vi "Reclosing.vi"(5 "Recloser Settings":T1, 6 "Counter In":dbl, 8 "Reclose In":bool, 9 "RMS values":dbl[](array[numeric]), 10 "PLL output":cluster{dbl, dbl[], dbl, dbl[]}, 11 "Reclose?":bool) -> (0 "Phase difference":dbl, 1 "frequency difference":dbl, 2 "magnitude difference":dbl, 3 "Recloser action":bool, 4 "Counter Out":dbl)   [LabVIEW 2016]
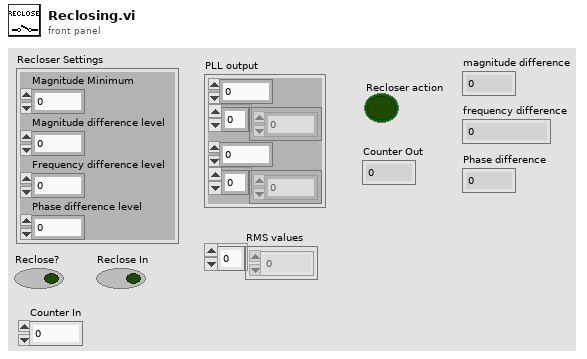
[diagram p1: front panel]
types:
  T1 = cluster{"Magnitude Minimum":dbl, "Magnitude difference level":dbl, "Frequency difference level":dbl, "Phase difference level":dbl}
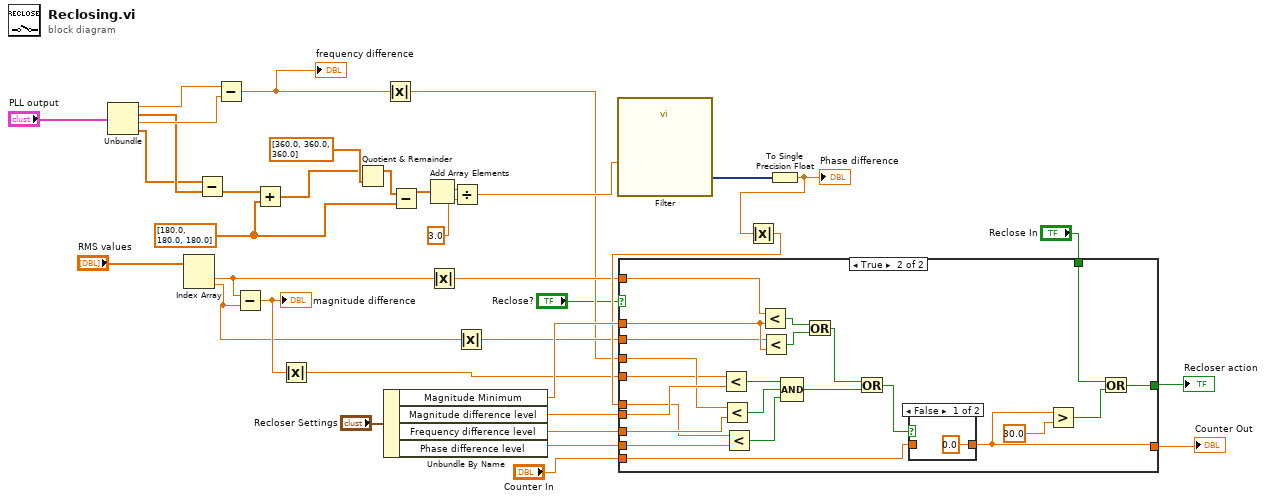
[diagram p0: block diagram]
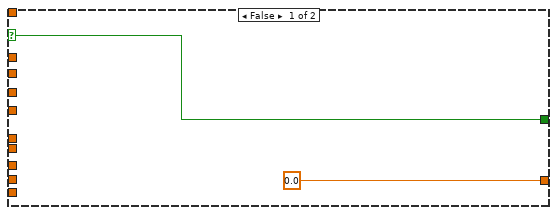
[diagram p2: hidden frame]
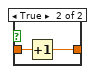
[diagram p3: hidden frame]
diagram:
  w26 = dbl[] [180.0, 180.0, 180.0] ("y")
  n1 = Unbundle("PLL output") -> (w14:dbl, w12:dbl[], w13:dbl, w11:dbl[])
  n2 = Index Array(array="RMS values") -> (element #1=w8:dbl, element #2=w7:dbl)  [unwired: 2 in]
  n3 = Subtract(x=w11, y=w12) -> (x-y=w36:dbl[])
  n4 = Subtract(x=w14, y=w13) -> (x-y=w10:dbl)
  "frequency difference" <- w10
  n5 = Subtract(x=w8, y=w7) -> (x-y=w20:dbl)
  "magnitude difference" <- w20
  n6 = Add(x=w36, y=w26) -> (x+y=w29:dbl[])
  n7 = Absolute Value(x=w20) -> (abs(x)=w2:dbl)
  n8 = Quotient & Remainder(x=w29, y=dbl[] [360.0, 360.0, 360.0]) -> (x-y*floor(x/y)=w32:dbl[])  [unwired: 1 out]
  n9 = Unbundle By Name("Recloser Settings") -> ("Magnitude Minimum"=w25:dbl, "Magnitude difference level"=w24:dbl, "Frequency difference level"=w23:dbl, "Phase difference level"=w22:dbl)
  n10 = Absolute Value(x=w10) -> (abs(x)=w16:dbl)
  n11 = Subtract(x=w32, y=w26) -> (x-y=w31:dbl[])
  n12 = Add Array Elements(numeric array=w31) -> (sum=w35:dbl)
  n13 = Absolute Value(x=w8) -> (abs(x)=w17:dbl)
  n14 = Divide(x=w35, y=3.0 ("x")) -> (x/y=w27:dbl)
  n15 = Absolute Value(x=w7) -> (abs(x)=w18:dbl)
  n16 = call "Filter"("Signal"=w27) -> ("Filtered Signal"=w30:dynamicdata)  [unwired: 9 in, 1 out]
  n17 = To Single Precision Float(number=w30) -> (single precision float=w21:sgl)
  "Phase difference" <- w21
  n18 = Absolute Value(x=w21) -> (abs(x)=w19:sgl)
  n19 = case shown="True" "Reclose?" {
    selector: "Reclose?" -> [w38 _]
    tunnel: [w38 w39] -> w3
    tunnel: [0.0 w43] -> w4
    tunnel: w25 -> [_ w54]
    tunnel: w24 -> [_ w53]
    tunnel: w23 -> [_ w52]
    tunnel: w22 -> [_ w51]
    tunnel: w19 -> [_ w50]
    tunnel: w16 -> [_ w49]
    tunnel: w2 -> [_ w48]
    tunnel: "Counter In" -> [_ w47]
    tunnel: w17 -> [_ w46]
    tunnel: w18 -> [_ w45]
    tunnel: "Reclose In" -> [_ w41]
    frame False {
    }
    frame True {
      n20 = Less?(x=w48, y=w53) -> (x < y?=w56:bool)
      n21 = Less?(x=w49, y=w52) -> (x < y?=w59:bool)
      n22 = Less?(x=w50, y=w51) -> (x < y?=w58:bool)
      n23 = Less?(x=w46, y=w54) -> (x < y?=w61:bool)
      n24 = Less?(x=w45, y=w54) -> (x < y?=w60:bool)
      n25 = Compound Arithmetic op=AND(w56, w59, w58) -> (w57:bool)
      n26 = Or(x=w61, y=w60) -> (x .or. y?=w55:bool)
      n27 = Or(x=w55, y=w57) -> (x .or. y?=w42:bool)
      n28 = case shown="False" w42 {
        tunnel: [0.0 w64] -> w43
        tunnel: w47 -> [_ w63]
        frame False {
        }
        frame True {
          n29 = Increment(x=w63) -> (x+1=w64:dbl)
        }
      }
      n30 = Greater?(x=w43, y=30.0 ("x")) -> (0:w40:bool)
      n31 = Or(x=w41, y=w40) -> (x .or. y?=w39:bool)
    }
  }
  "Recloser action" <- w3
  "Counter Out" <- w4
